vi "test.vi"() -> ()   [LabVIEW 2018]
uses:
  <vilib>/Utility/file.llb/Write Delimited Spreadsheet (DBL).vi
panel:
  out "x+1":dbl[](array[numeric])
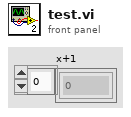
[diagram p1: front panel]
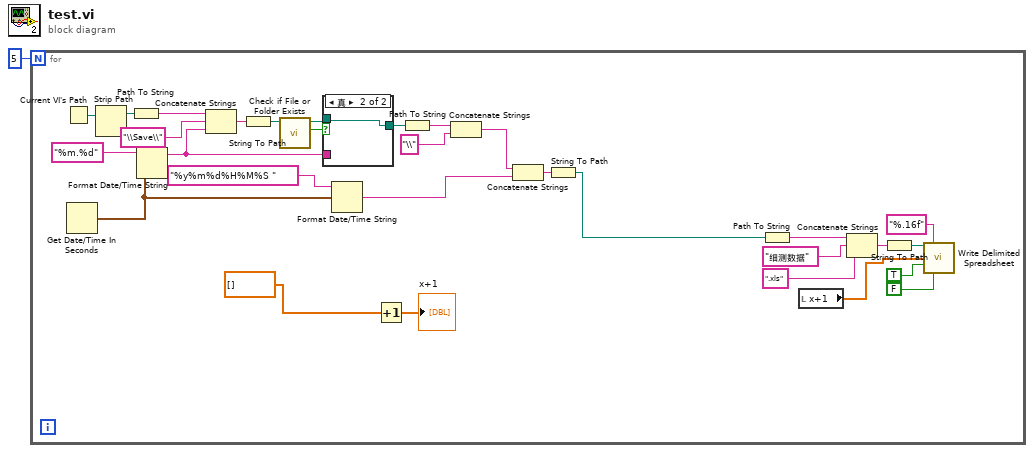
[diagram p0: block diagram]
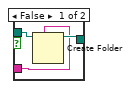
[diagram p2: hidden frame]
diagram:
  n1 = for {
    N: 5 -> [_]
    n2 = Current VI's Path() -> (path=w12:path)
    n3 = Get Date/Time In Seconds() -> (seconds since 1Jan1904=w6:timestamp)
    n4 = Strip Path(path=w12) -> (stripped path=w13:path)  [unwired: 1 out]
    n5 = Path To String(path=w13) -> (string=w14:string)
    n6 = Format Date/Time String(time format string (%c)="%m.%d" ("时间格式字符串(%c)"), seconds (now)=w6) -> (date/time string=w20:string)  [unwired: 1 in]
    n7 = Concatenate Strings(w14, "\\Save\\" ("字符串"), w20) -> (w15:string)
    n8 = String To Path(string=w15) -> (path=w16:path)
    n9 = call <vilib>:"Check if File or Folder Exists.vi"("path"=w16) -> ("file or folder exists?"=w17:bool, "dup path"=w19:path)  [unwired: 8 in, 1 out]
    n10 = case shown="真" w17 {
      tunnel: [w34 w35] -> w18
      tunnel: w19 -> [w33 w35]
      tunnel: w20 -> [w32 _]
      frame False {
        n11 = Create Folder(prompt (Create Folder)=w32, path (use dialog)=w33) -> (created path=w34:path)  [unwired: 1 in, 2 out]
      }
      frame True {
      }
    }
    n12 = Format Date/Time String(time format string (%c)="%y%m%d%H%M%S " ("时间格式字符串(%c)"), seconds (now)=w6) -> (date/time string=w23:string)  [unwired: 1 in]
    n13 = Increment(x=dbl[] []) -> (x+1=→"x+1":dbl[])
    n14 = Path To String(path=w18) -> (string=w21:string)
    n15 = Concatenate Strings(w21, "\\" ("字符串")) -> (w22:string)
    n16 = Concatenate Strings(w22, w23) -> (w11:string)
    n17 = String To Path(string=w11) -> (path=w5:path)
    n18 = Path To String(path=w5) -> (string=w31:string)
    n19 = local read "x+1"() -> (w2:dbl[])
    n20 = Concatenate Strings(w31, "细测数据" ("字符串"), ".xls" ("字符串")) -> (w24:string)
    n21 = String To Path(string=w24) -> (path=w30:path)
    n22 = call-poly <vilib>:"Write Delimited Spreadsheet.vi"("file path (dialog if empty)"=w30, "format (%.3f)"="%.16f", "1D data"=w2, "append to file? (new file:F)"=TRUE ("append to file? (F)"), "transpose? (no:F)"=FALSE ("transpose? (F)")) -> ()  [unwired: 9 in, 2 out]
  }
